vi "test_NEO480HTA get all data.vi"(8 "Error In":errorcluster) -> (0 "Error Out":errorcluster)   [LabVIEW 2024]
uses:
  Real All CFG/Read All CFG.lvclass
  MSS/MSS.lvclass
panel:
  out "i":i32
  out "Absolute Humidity":dbl format="%#_g g m^-3"
  out "Pressure":dbl format="%#_g mbar"
  out "Dew Point":dbl format="%#_g °C"
  out "Temperature":dbl format="%#_g °C"
  in  "Stop":bool
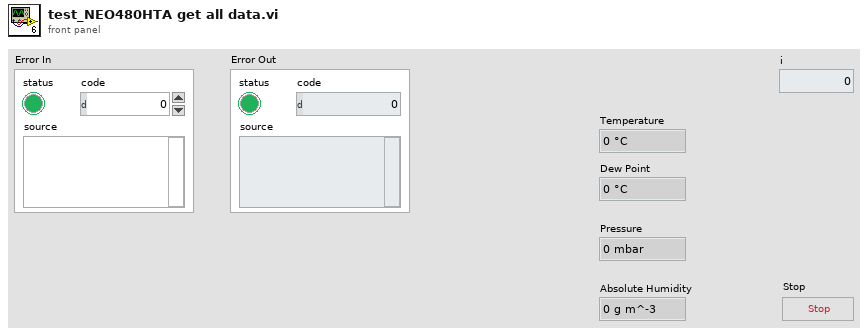
[diagram p1: front panel]
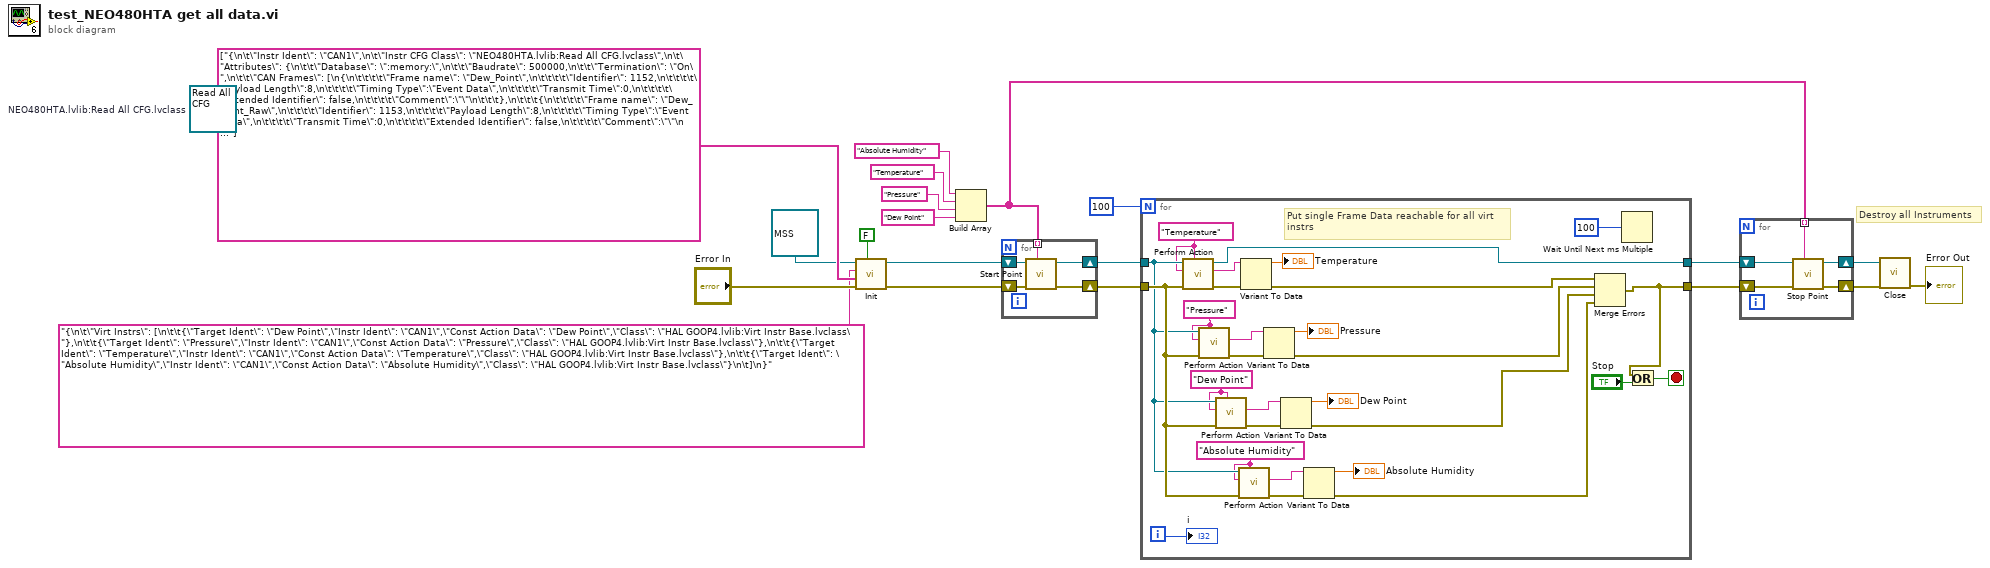
[diagram p0: block diagram]
diagram:
  (unwired) refnum<class "Read All CFG.lvclass"> refnum  # NEO480HTA.lvlib:Read All CFG.lvclass
  # "Destroy all Instruments"
  n1 = call "Init.vi"("Is Target?"=FALSE, "error in"="Error In", "Instr CFGs"=string[] ["{\n\t\"Instr Ident\": \"CAN1\",\n\t\"Instr CFG Class\": \"NEO480HTA.lvlib:Read All CFG.lvclass\",\n\t\"Attributes\": {\n\t\t\"Database\": \":memory:\",\n\t\t\"Baudrate\": 500000,\n\t\t\"Termination\": \"On\",\n\t\t\"CAN Frames\": [\n{\n\t\t\t\t\"Frame name\": \"Dew_Point\",\n\t\t\t\t\"Identifier\": 1152,\n\t\t\t\t\"Payload Length\":8,\n\t\t\t\t\"Timing Type\":\"Event Data\",\n\t\t\t\t\"Transmit Time\":0,\n\t\t\t\t\"Extended Identifier\": false,\n\t\t\t\t\"Comment\":\"\"\n\t\t\t},\n\t\t\t{\n\t\t\t\t\"Frame name\": \"Dew_Point_Raw\",\n\t\t\t\t\"Identifier\": 1153,\n\t\t\t\t\"Payload Length\":8,\n\t\t\t\t\"Timing Type\":\"Event Data\",\n\t\t\t\t\"Transmit Time\":0,\n\t\t\t\t\"Extended Identifier\": false,\n\t\t\t\t\"Comment\":\"\"\n                      }\n],\n\t\t\"Acquire\": {\n\t\t\t\"Type\": \"Read Frame\"\n\t\t}\n\t}\n}"], "<JSON> Virt Instr CFG"="{\n\t\"Virt Instrs\": [\n\t\t{\"Target Ident\": \"Dew Point\",\"Instr Ident\": \"CAN1\",\"Const Action Data\": \"Dew Point\",\"Class\": \"HAL GOOP4.lvlib:Virt Instr Base.lvclass\"},\n\t\t{\"Target Ident\": \"Pressure\",\"Instr Ident\": \"CAN1\",\"Const Action Data\": \"Pressure\",\"Class\": \"HAL GOOP4.lvlib:Virt Instr Base.lvclass\"},\n\t\t{\"Target Ident\": \"Temperature\",\"Instr Ident\": \"CAN1\",\"Const Action Data\": \"Temperature\",\"Class\": \"HAL GOOP4.lvlib:Virt Instr Base.lvclass\"},\n\t\t{\"Target Ident\": \"Absolute Humidity\",\"Instr Ident\": \"CAN1\",\"Const Action Data\": \"Absolute Humidity\",\"Class\": \"HAL GOOP4.lvlib:Virt Instr Base.lvclass\"}\n\t]\n}", "MSS in"=refnum<class "MSS.lvclass"> refnum) -> ("error out"=w15:errorcluster, "MSS out"=w14:refnum<class "MSS.lvclass">)  [unwired: 3 in, 2 out]
  n2 = Build Array("Absolute Humidity" ("Target Ident"), "Temperature" ("Target Ident"), "Pressure" ("Target Ident"), "Dew Point" ("Target Ident")) -> (w4:string[])
  n3 = for {
    shift-right: [w25] -> w17
    shift-left: w15 -> [w24]
    shift-right: [w22] -> w13
    shift-left: w14 -> [w23]
    tunnel: w4 -> [w21] mode=indexing
    n4 = call "Start Point.vi"("Task-Point Ident"=w21, "error in"=w24, "MSS in"=w23) -> ("error out"=w25:errorcluster, "MSS out"=w22:refnum<class "MSS.lvclass">)  [unwired: 7 in]
  }
  n5 = for {
    N: 100 -> [_]
    tunnel: w17 -> [w40]
    tunnel: w13 -> [w39]
    tunnel: [w37] -> w5
    tunnel: [w34] -> w6
    i -> [w30]
    stop <- w53 stop-if-true
    w28 = "Absolute Humidity" ("Target Identifier")
    w29 = "Dew Point" ("Target Identifier")
    w26 = "Temperature" ("Target Identifier")
    w27 = "Pressure" ("Target Identifier")
    # "Put single Frame Data reachable for all virt\ninstrs"
    n6 = call "Perform Action.vi"("Task Ident"=w26, "error in"=w40, "Point Ident"=w26, "MSS in"=w39) -> ("error out"=w49:errorcluster, "Task-Point Ident"=w48:string, "MSS out"=w37:refnum<class "MSS.lvclass">)  [unwired: 4 in, 1 out]
    n7 = call "Perform Action.vi"("Task Ident"=w27, "error in"=w40, "Point Ident"=w27, "MSS in"=w39) -> ("error out"=w51:errorcluster, "Task-Point Ident"=w50:string)  [unwired: 4 in, 2 out]
    n8 = call "Perform Action.vi"("Task Ident"=w29, "error in"=w40, "Point Ident"=w29, "MSS in"=w39) -> ("error out"=w45:errorcluster, "Task-Point Ident"=w44:string)  [unwired: 4 in, 2 out]
    n9 = call "Perform Action.vi"("Task Ident"=w28, "error in"=w40, "Point Ident"=w28, "MSS in"=w39) -> ("error out"=w41:errorcluster, "Task-Point Ident"=w42:string)  [unwired: 4 in, 2 out]
    n10 = Variant To Data(error in=w49, Variant=w48) -> (data=→"Temperature":dbl, error out=w36:errorcluster)  [unwired: 1 in]
    n11 = Variant To Data(error in=w51, Variant=w50) -> (data=→"Pressure":dbl, error out=w35:errorcluster)  [unwired: 1 in]
    n12 = Variant To Data(error in=w45, Variant=w44) -> (data=→"Dew Point":dbl, error out=w33:errorcluster)  [unwired: 1 in]
    n13 = Variant To Data(error in=w41, Variant=w42) -> (data=→"Absolute Humidity":dbl, error out=w32:errorcluster)  [unwired: 1 in]
    n14 = Merge Errors(w36, w35, w33, w32) -> (w34:errorcluster)
    n15 = Wait Until Next ms Multiple(millisecond multiple=u32 100) -> ()  [unwired: 1 out]
    n16 = Or(x=w34, y="Stop") -> (x .or. y?=w53:bool)
    "i" <- w30
  }
  n17 = for {
    shift-right: [w57] -> w7
    shift-left: w6 -> [w56]
    shift-right: [w58] -> w8
    shift-left: w5 -> [w55]
    tunnel: w4 -> [w54] mode=indexing
    n18 = call "Stop Point.vi"("Task-Point Ident"=w54, "error in"=w56, "MSS in"=w55) -> ("error out"=w57:errorcluster, "MSS out"=w58:refnum<class "MSS.lvclass">)  [unwired: 7 in]
  }
  n19 = call "Close.vi"("error in"=w7, "MSS in"=w8) -> ("error out"=→"Error Out":errorcluster)  [unwired: 8 in, 1 out]
